vi "Calclulator-Add.vi"(10 "y":dbl, 11 "x":dbl) -> (3 "x plus y":dbl)   [LabVIEW 2025]
doc: "adds two numbers"
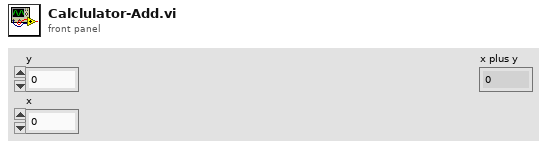
[diagram p1: front panel]
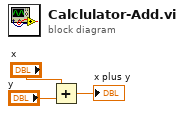
[diagram p0: block diagram]
diagram:
  n1 = Add(x="x", y="y") -> (x+y=→"x plus y":dbl)
